vi "Remove and Unmap Output Channel.vi"(8 "error in (no error)":errorcluster, 9 "Channel Name":string, 10 "engine":refnum<data-value>, 11 "E2E editor node in":refnum<data-value>) -> (0 "error out":errorcluster, 2 "engine out":refnum<data-value>, 3 "E2E editor node out":refnum<data-value>)   [LabVIEW 2015, in "E2E Tag Exchange editor node.lvclass"]
uses:
  E2E Tag Exchange editor node.lvclass
  <vilib>/NI/DCAF/Tag Editor Core/Configuration Editor/Classes/Engine Parent/Engine Parent Editor Node.lvclass
  E2E Tag Exchange editor node.lvclass/E2E Tag Exchange editor node.ctl
  <vilib>/NI/Configuration Framework/serializable configuration/NISE_CEF_serializable configuration.lvclass/NISE_CEF_serializable configuration.ctl
  <vilib>/Utility/LVClass/Get LV Class Name.vi
  <vilib>/NI/Configuration Framework/error generator/NISE_error generator.vi
  <vilib>/NI/Configuration Framework/serializable configuration/NISE_CEF_serializable configuration.lvclass
  module/configuration/E2E Tag Exchange configuration.lvclass
  <vilib>/NI/Module Execution Interface/Engine Configuration/engine configuration.lvclass
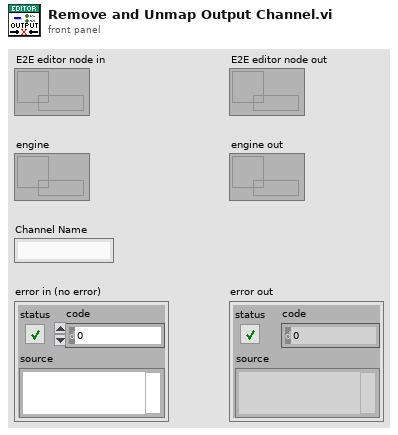
[diagram p1: front panel]
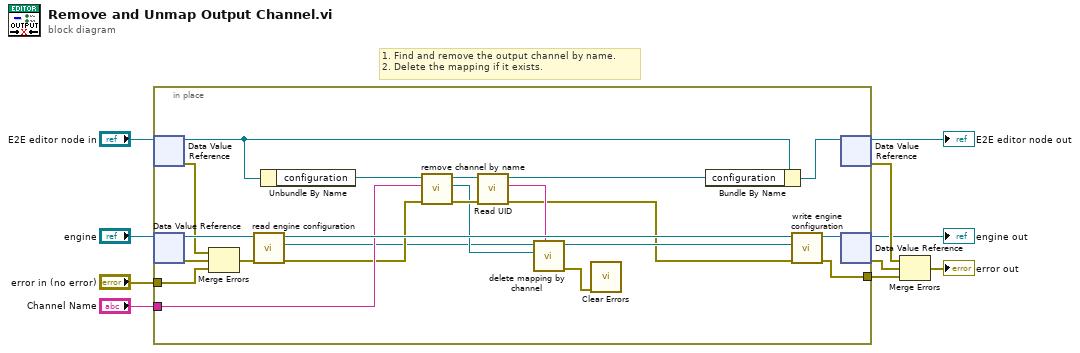
[diagram p0: block diagram]
diagram:
  # "1. Find and remove the output channel by name.\n2. Delete the mapping if it exists."
  n1 = in-place {
    in-place-border: "Channel Name" -> [w17]
    in-place-border: "error in (no error)" -> [w22]
    in-place-border: [w18] -> w6
    n2 = in-place-dvr #1("E2E editor node in") -> (w27:refnum<class "E2E Tag Exchange editor node.lvclass">, w19:errorcluster)
    n3 = in-place-dvr #2("engine") -> (w32:refnum<class "Engine Parent Editor Node.lvclass">, w21:errorcluster)
    n4 = Merge Errors(w19, w21, w22) -> (w20:errorcluster)
    n5 = call <vilib>:"read engine configuration.vi"("error in"=w20, "Engine Parent Editor Node in"=w32) -> ("error out"=w12:errorcluster, "engine configuration"=w11:refnum<class "engine configuration.lvclass">, "Engine Parent Editor Node out"=w24:refnum<class "Engine Parent Editor Node.lvclass">)  [unwired: 7 in]
    n6 = Unbundle By Name(w27) -> ("configuration"=w31:refnum<class "E2E Tag Exchange configuration.lvclass">)
    n7 = call "remove channel by name.vi"("error in (no error)"=w12, "name"=w17, "E2E configuration in"=w31) -> ("error out"=w29:errorcluster, "removed channel"=w15:refnum<class "TBM channel.lvclass">, "E2E configuration out"=w30:refnum<class "E2E Tag Exchange configuration.lvclass">)  [unwired: 6 in]
    n8 = call <vilib>:"Read UID.vi"("error in"=w29, "configuration in"=w30) -> ("error out"=w13:errorcluster, "instance id"=w16:string, "configuration out"=w28:refnum<class "E2E Tag Exchange configuration.lvclass">)  [unwired: 7 in]
    n9 = call <vilib>:"delete mapping by channel.vi"("owner ID"=w16, "channel"=w15, "engine configuration in"=w11) -> ("error out"=w14:errorcluster, "engine configuration out"=w23:refnum<class "engine configuration.lvclass">)  [unwired: 7 in]
    n10 = call <vilib>:"Clear Errors.vi"("error in (no error)"=w14) -> ()  [unwired: 5 in, 2 out]
    n11 = Bundle By Name(cluster=w27, "configuration"=w28) -> (w26:refnum<class "E2E Tag Exchange editor node.lvclass">)
    n12 = call <vilib>:"write engine configuration.vi"("error in"=w13, "engine configuration"=w23, "Engine Parent Editor Node in"=w24) -> ("error out"=w18:errorcluster, "Engine Parent Editor Node out"=w25:refnum<class "Engine Parent Editor Node.lvclass">)  [unwired: 7 in]
    n13 = in-place-dvr #1(w26) -> (→"E2E editor node out":refnum<data-value>, w4:errorcluster)
    n14 = in-place-dvr #2(w25) -> (→"engine out":refnum<data-value>, w5:errorcluster)
  }
  n15 = Merge Errors(w4, w5, w6) -> (→"error out":errorcluster)
